vi "Queue Driver.vi"(0 "Queue Name":string, 2 "States[]":string[](array[string]), 11 "error In":errorcluster, 13 "Queue Operation":T1) -> (4 "Dequeued State":string, 15 "error out":errorcluster)   [LabVIEW 2016]
uses:
  Typedef/Queue Operation.ctl
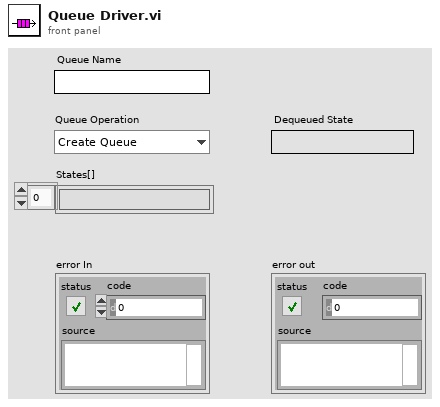
[diagram p1: front panel]
types:
  T1 = typedef "Queue Operation.ctl" = enum16{"Create Queue", "Enqueue N Element", "Enstack N Element", "Dequeue 1 Element", "Flush Queue", "Close Queue"}
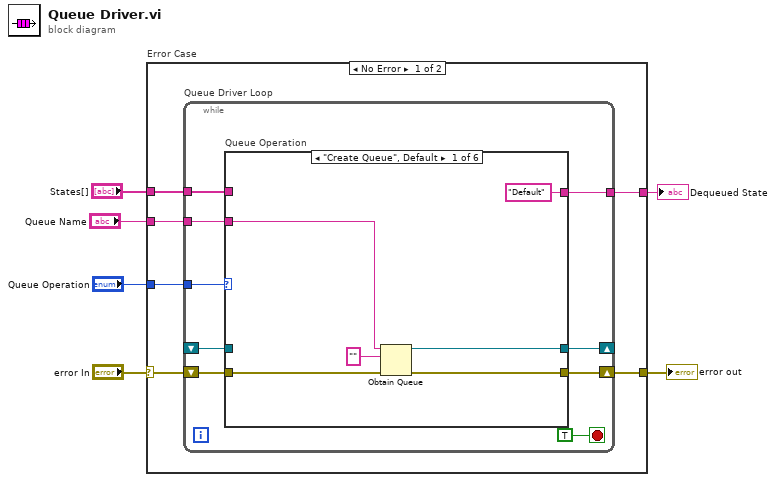
[diagram p0: block diagram]
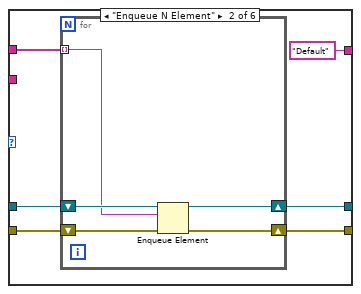
[diagram p2: hidden frame]
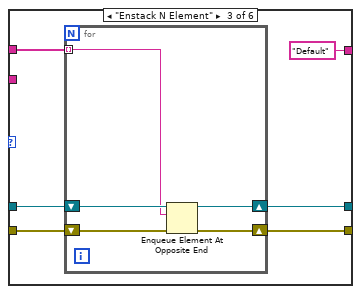
[diagram p3: hidden frame]
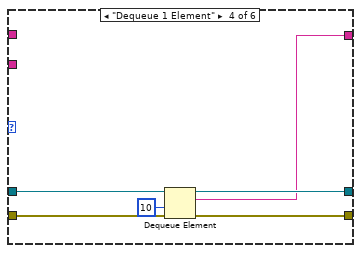
[diagram p4: hidden frame]
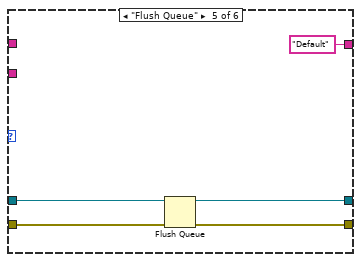
[diagram p5: hidden frame]
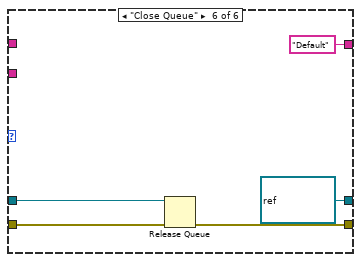
[diagram p6: hidden frame]
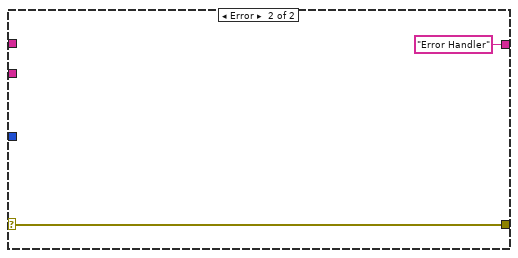
[diagram p7: hidden frame]
diagram:
  n1 = case "Error Case" shown="No Error" "error In" {
    selector: "error In" -> [w12 w67]
    tunnel: [w11 w67] -> w5
    tunnel: "Queue Operation" -> [w10 _]
    tunnel: "States[]" -> [w9 _]
    tunnel: "Queue Name" -> [w8 _]
    tunnel: [w7 "Error Handler"] -> w1
    frame No Error {
      n2 = while "Queue Driver Loop" {
        shift-right: [w19] -> w11
        shift-left: w12 -> [w20]
        tunnel: w10 -> [w18]
        tunnel: w9 -> [w17]
        tunnel: w8 -> [w16]
        shift-right: [w15] -> _
        shift-left: _ -> [w14]
        tunnel: [w13] -> w7
        stop <- TRUE stop-if-true
        n3 = case "Queue Operation" shown="\"Create Queue\", Default" w18 {
          tunnel: w20 -> [w27 w33 w44 w55 w60 w65]
          tunnel: [w26 w32 w43 w54 w59 w64] -> w19
          tunnel: w17 -> [_ w29 w40 _ _ _]
          tunnel: w16 -> [w25 _ _ _ _ _]
          tunnel: [w24 w30 w41 w51 w57 refnum<queue> refnum ("queue out")] -> w15
          tunnel: w14 -> [_ w31 w42 w53 w58 w63]
          tunnel: ["Default" "Default" "Default" w50 "Default" "Default"] -> w13
          frame "Create Queue", Default {
            n4 = Obtain Queue(name (unnamed)=w25, element data type="", error in (no error)=w27) -> (queue out=w24:refnum<queue>, error out=w26:errorcluster)  [unwired: 2 in, 1 out]
          }
          frame "Enqueue N Element" {
            n5 = for {
              shift-right: [w37] -> w32
              shift-left: w33 -> [w38]
              shift-right: [w35] -> w30
              shift-left: w31 -> [w36]
              tunnel: w29 -> [w34] mode=indexing
              n6 = Enqueue Element(queue=w36, element=w34, error in (no error)=w38) -> (queue out=w35:refnum<queue>, error out=w37:errorcluster)  [unwired: 1 in, 1 out]
            }
          }
          frame "Enstack N Element" {
            n7 = for {
              shift-right: [w48] -> w43
              shift-left: w44 -> [w49]
              shift-right: [w46] -> w41
              shift-left: w42 -> [w47]
              tunnel: w40 -> [w45] mode=indexing
              n8 = Enqueue Element At Opposite End(queue=w47, element=w45, error in (no error)=w49) -> (queue out=w46:refnum<queue>, error out=w48:errorcluster)  [unwired: 1 in, 1 out]
            }
          }
          frame "Dequeue 1 Element" {
            n9 = Dequeue Element(queue=w53, timeout in ms (-1)=10, error in (no error)=w55) -> (queue out=w51:refnum<queue>, element=w50:string, error out=w54:errorcluster)  [unwired: 1 out]
          }
          frame "Flush Queue" {
            n10 = Flush Queue(queue=w58, error in (no error)=w60) -> (queue out=w57:refnum<queue>, error out=w59:errorcluster)  [unwired: 1 out]
          }
          frame "Close Queue" {
            n11 = Release Queue(queue=w63, error in (no error)=w65) -> (error out=w64:errorcluster)  [unwired: 1 in, 2 out]
          }
        }
      }
    }
    frame Error {
    }
  }
  "Dequeued State" <- w1
  "error out" <- w5
